vi "SetPPMSField.vi"(0 "Approach":dbl, 1 "Mode":dbl=1.0, 2 "Rate":dbl=10.0, 3 "Field":dbl=300.0) -> ()   [LabVIEW 2013]
uses:
  C:/QdLabview/QDInstrument.dll
panel:
  in  "Instrument\nType 2":i32(ring) items=["PPMS", "VersaLab", "DynaCool", "SVSM"]
  in  "Remote 2":bool
  in  "IP Address 2":string="127.0.0.1"
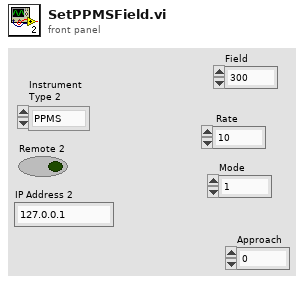
[diagram p1: front panel]
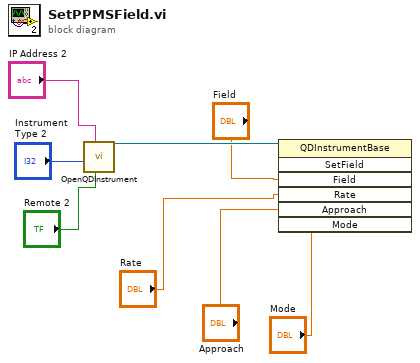
[diagram p0: block diagram]
diagram:
  n1 = call "OpenQDInstrument.vi"("Remote"="Remote 2", "IP Address"="IP Address 2", "Instrument Type"="Instrument\nType 2") -> ("Instrument Ref"=w5:refnum<k24>)  [unwired: 5 in, 1 out]
  n2 = invoke class="QDInstrumentBase" method="SetField"(reference=w5, "Field"="Field", "Rate"="Rate", "Approach"="Approach", "Mode"="Mode") -> ()  [unwired: 2 in, 7 out]
